vi "Create Pattern Script(Data).vi"(8 "error in (no error)":errorcluster, 11 "Data":u8[](array[numeric])) -> (0 "error out":errorcluster, 3 "String":string)   [LabVIEW 2018, in "BML_Frame_Root.lvclass"]
uses:
  BML_Frame_Root.lvclass
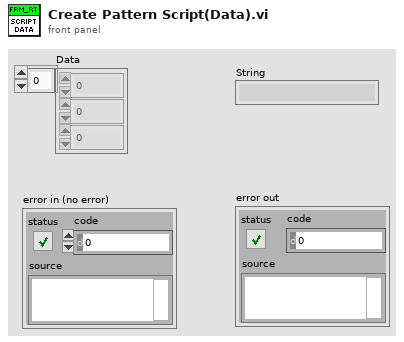
[diagram p1: front panel]
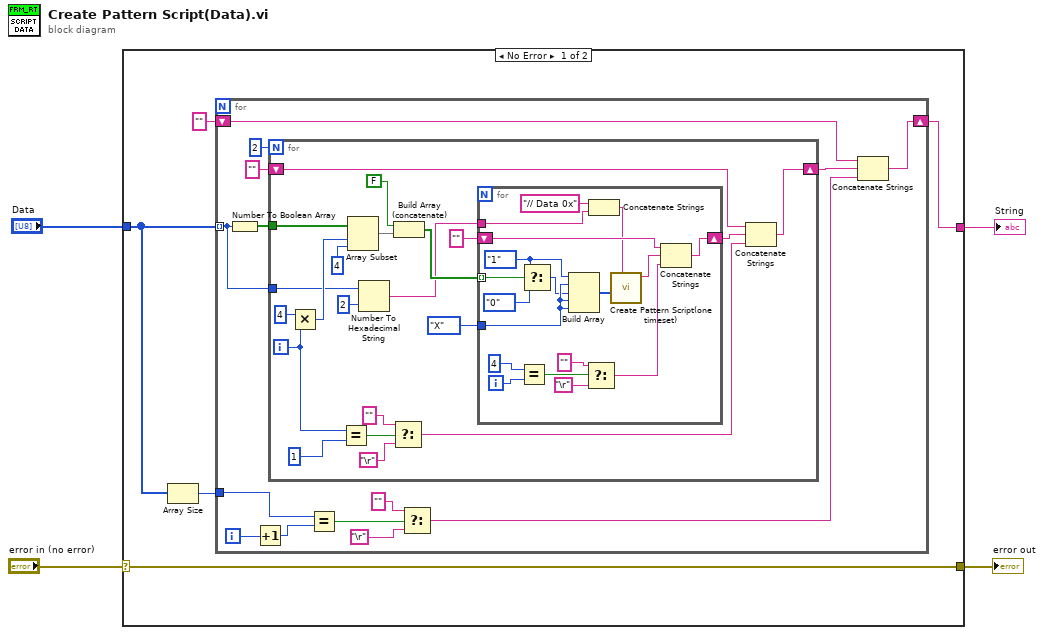
[diagram p0: block diagram]
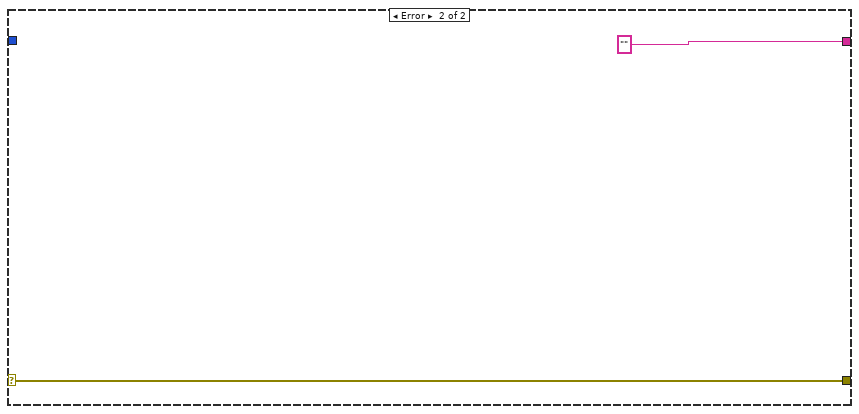
[diagram p2: hidden frame]
diagram:
  n1 = case shown="No Error" "error in (no error)" {
    selector: "error in (no error)" -> [w9 w63]
    tunnel: [w6 ""] -> w3
    tunnel: [w9 w63] -> w2
    tunnel: "Data" -> [w8 _]
    frame No Error {
      n2 = Array Size(array=w8) -> (size(s)=w7:i32)
      n3 = for {
        tunnel: w8 -> [w10] mode=indexing
        tunnel: w7 -> [w18]
        shift-right: [w12] -> w6
        shift-left: "" -> [w11]
        i -> [w20]
        n4 = Number To Boolean Array(number=w10) -> (Boolean array=w23:bool[])
        n5 = Increment(x=w20) -> (x+1=w19:i32)
        n6 = for {
          N: 2 -> [_]
          tunnel: w23 -> [w44]
          shift-right: [w30] -> w14
          shift-left: "" -> [w29]
          tunnel: w10 -> [w26]
          i -> [w37]
          n7 = Multiply(x=4 ("y"), y=w37) -> (x*y=w43:i32)
          n8 = Equal?(x=w37, y=1) -> (x = y?=w35:bool)
          n9 = Array Subset(array=w44, index=w43, length=4) -> (w42:bool[])
          n10 = Number To Hexadecimal String(1:i16 2 ("width (-)"), 2:w26) -> (0:w24:string)
          n11 = Select(t="", s=w35, f="\r") -> (s? t:f=w31:string)
          n12 = Build Array (concatenate)(FALSE, w42) -> (w39:bool[])
          n13 = for {
            tunnel: w39 -> [w62] mode=indexing
            shift-right: [w55] -> w32
            shift-left: "" -> [w54]
            tunnel: enum16{"0", "1", "L", "H", "X", "V", "D", "M"}."X" ("element") -> [w52]
            tunnel: w24 -> [w46]
            i -> [w60]
            w49 = enum16{"0", "1", "L", "H", "X", "V", "D", "M"}."1" ("PinState")
            n14 = Equal?(x=4, y=w60) -> (x = y?=w58:bool)
            n15 = Select(t=w49, s=w62, f=enum16{"0", "1", "L", "H", "X", "V", "D", "M"}."0") -> (s? t:f=w48:enum16{"0", "1", "L", "H", "X", "V", "D", "M"})
            n16 = Build Array(w49, w52, w48, w52, w52) -> (w51:enum16{"0", "1", "L", "H", "X", "V", "D", "M"}[])
            n17 = Select(t="", s=w58, f="\r") -> (s? t:f=w53:string)
            n18 = Concatenate Strings("// Data 0x" ("string"), w46) -> (w45:string)
            n19 = call "Create Pattern Script(one timeset).vi"("Notes"=w45, "PinState"=w51) -> ("string out"=w50:string)  [unwired: 9 in]
            n20 = Concatenate Strings(w54, w50, w53) -> (w55:string)
          }
          n21 = Concatenate Strings(w29, w32, w31) -> (w30:string)
        }
        n22 = Equal?(x=w18, y=w19) -> (x = y?=w15:bool)
        n23 = Select(t="", s=w15, f="\r") -> (s? t:f=w13:string)
        n24 = Concatenate Strings(w11, w14, w13) -> (w12:string)
      }
    }
    frame Error {
    }
  }
  "String" <- w3
  "error out" <- w2
